vi "display.vi"(8 "error in (no error)":errorcluster, 10 "GridRepresentable.lvclass":refnum<class "GridRepresentable.lvclass">, 11 "AbstractMultiColumnListBoxAdapter in":refnum<class "AbstractMultiColumnListBoxAdapter.lvclass">) -> (0 "error out":errorcluster, 3 "AbstractMultiColumnListBoxAdapter out":refnum<class "AbstractMultiColumnListBoxAdapter.lvclass">)   [LabVIEW 2020, in "AbstractMultiColumnListBoxAdapter.lvclass"]
uses:
  AbstractMultiColumnListBoxAdapter.lvclass
  GridDisplayable/GridRepresentable.lvclass
  AbstractMultiColumnListBoxAdapter.lvclass/AbstractMultiColumnListBoxAdapter.ctl
  <vilib>/Utility/miscctls.llb/LVRowAndColumnTypeDef.ctl
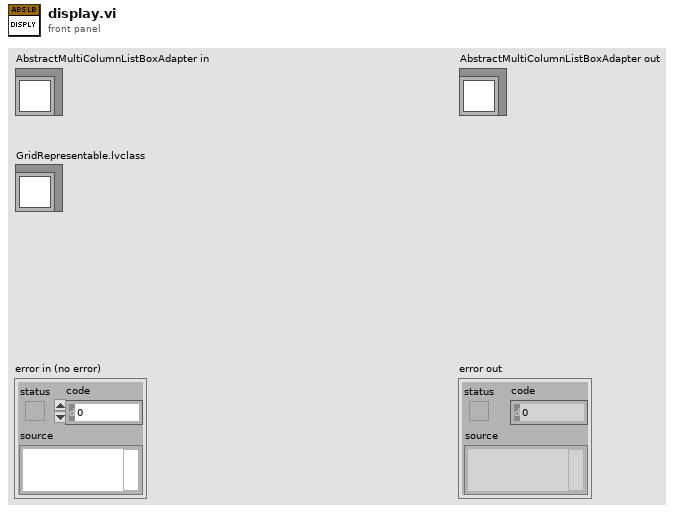
[diagram p1: front panel]
types:
  T1 = typedef "LVRowAndColumnTypeDef.ctl" = cluster{"Row":i32, "Column":i32}
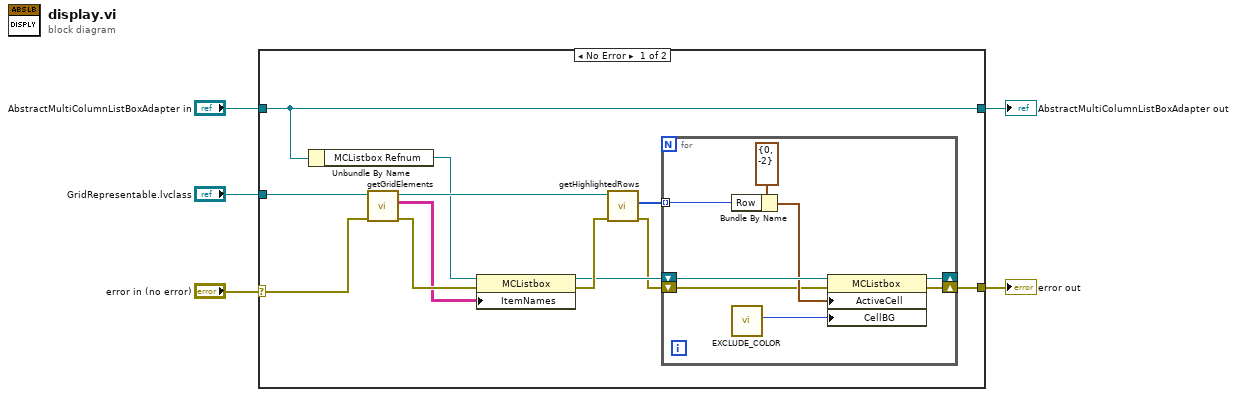
[diagram p0: block diagram]
diagram:
  n1 = case shown="No Error" "error in (no error)" {
    selector: "error in (no error)" -> [w15 w27]
    tunnel: [w7 w27] -> w4
    tunnel: [w14 w26] -> w2
    tunnel: "AbstractMultiColumnListBoxAdapter in" -> [w14 w26]
    tunnel: "GridRepresentable.lvclass" -> [w17 _]
    frame No Error {
      n2 = Unbundle By Name(w14) -> ("MCListbox Refnum"=w13:refnum<vi>)
      n3 = call-dynamic "getGridElements.vi"("error in (no error)"=w15, "GridDisplayable in"=w17) -> ("error out"=w12:errorcluster, "Grid Rows"=w10:string[][], "GridDisplayable out"=w16:refnum<class "GridRepresentable.lvclass">)  [unwired: 7 in]
      n4 = property class="MCListbox"(reference=w13, error in=w12, "ItemNames"=w10) -> (reference out=w8:refnum<vi>, error out=w11:errorcluster)
      n5 = call-dynamic "getHighlightedRows.vi"("error in (no error)"=w11, "GridDisplayable in"=w16) -> ("error out"=w6:errorcluster, "Highlighted Rows"=w9:i32[])  [unwired: 7 in, 1 out]
      n6 = for {
        tunnel: w9 -> [w21] mode=indexing
        shift-right: [w25] -> _
        shift-left: w8 -> [w24]
        shift-right: [w23] -> w7
        shift-left: w6 -> [w19]
        n7 = Bundle By Name(cluster=T1 {"Row"=0, "Column"=-2} ("Active Cell:Active Cell"), "Row"=w21) -> (w20:T1)
        n8 = call "EXCLUDE_COLOR.vi"() -> ("Color Box"=w18:u32)  [unwired: 11 in]
        n9 = property class="MCListbox"(reference=w24, error in=w19, "ActiveCell"=w20, "CellBG"=w18) -> (reference out=w25:refnum<vi>, error out=w23:errorcluster)
      }
    }
    frame Error {
    }
  }
  "error out" <- w4
  "AbstractMultiColumnListBoxAdapter out" <- w2
